vi "get_frekans_value_1D_array.vi"(9 "LstBox Refnum":refnum<vi>, 10 "frekans":dbl, 11 "F Values Array":dbl[][](array[numeric])) -> (2 "symbol enable?":i32, 3 "output array":dbl[](array[numeric]))   [LabVIEW 2014]
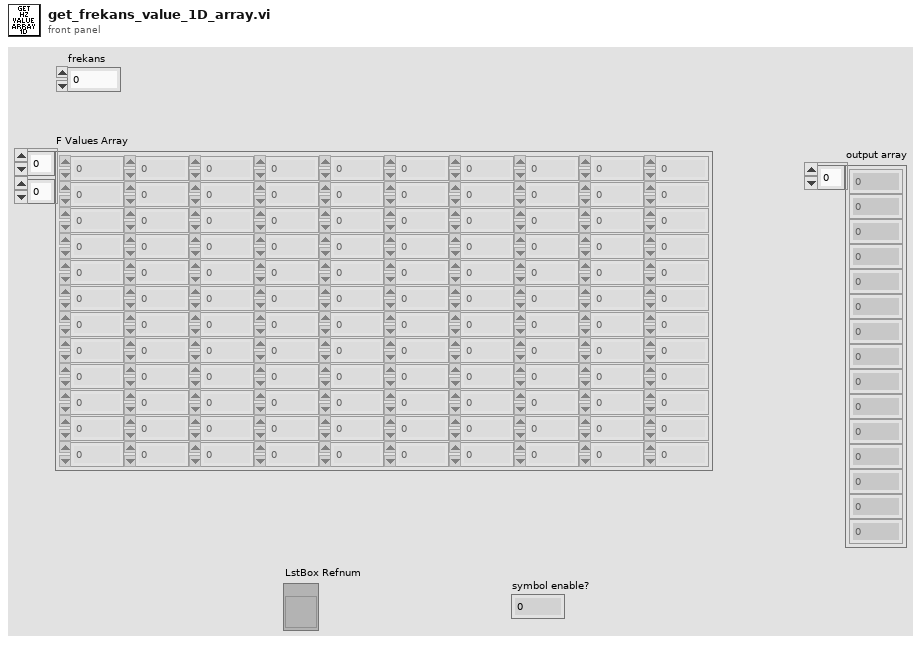
[diagram p1: front panel]
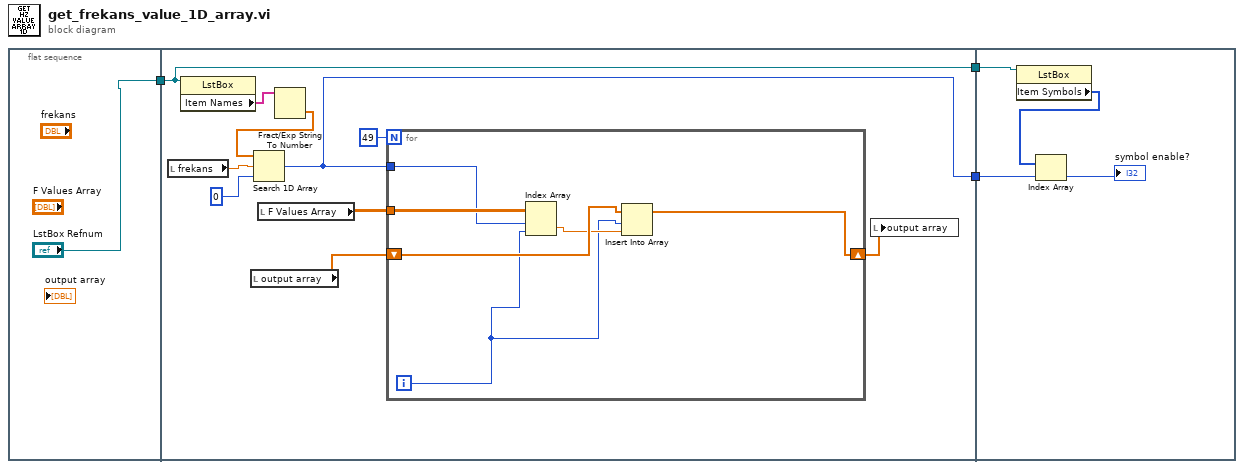
[diagram p0: block diagram]
diagram:
  n1 = flat-sequence {
    tunnel: ["LstBox Refnum"] -> w2
    tunnel: [w8] -> w3
    tunnel: w2 -> [w6]
    tunnel: [w6] -> w1
    tunnel: w3 -> [w24]
    tunnel: w1 -> [w22]
    frame #0 {
    }
    frame #1 {
      n2 = local read "frekans"() -> (w10:dbl)
      n3 = property class="LstBox"(reference=w6) -> ("Item Names"=w7:string[])  [unwired: 1 in, 2 out]
      n4 = local read "output array"() -> (w13:dbl[])
      n5 = local read "F Values Array"() -> (w12:dbl[][])
      n6 = Fract/Exp String To Number(string=w7) -> (number=w9:dbl[])  [unwired: 3 in, 1 out]
      n7 = Search 1D Array(1D array=w9, element=w10, start index (0)=0) -> (index of element=w8:i32)
      n8 = for {
        N: 49 -> [_]
        shift-right: [w17] -> w11
        shift-left: w13 -> [w19]
        tunnel: w12 -> [w20]
        tunnel: w8 -> [w16]
        i -> [w15]
        n9 = Index Array(array=w20, index (row)=w16, index (col)=w15) -> (element=w18:dbl)
        n10 = Insert Into Array(array=w19, index=w15, new element=w18) -> (w17:dbl[])
      }
      n11 = local write "output array"(w11) -> ()
    }
    frame #2 {
      n12 = property class="LstBox"(reference=w22) -> ("Item Symbols"=w21:i32[])  [unwired: 1 in, 2 out]
      n13 = Index Array(array=w21, index=w24) -> (element=→"symbol enable?":i32)
    }
  }
